vi "BNC555.ProcCases.vi"(0 "i ref in":refnum<vi>, 1 "selector":string, 2 "data":i8[](array[numeric]), 3 "call cluster":T1={"Object"="", "Selector"="", "CallType"=enum."synchronous", "Async Object"="", "Async Selector"="", "Data Descriptor"="", "Data"=[], "Error #"=0, "Expire"=0}, 5 "error in":errorcluster) -> (14 "i ref out":refnum<vi>, 17 "answer cluster":T1={"Object"="", "Selector"="", "CallType"=enum."synchronous", "Async Object"="", "Async Selector"="", "Data Descriptor"="", "Data"=[], "Error #"=0, "Expire"=0}, 19 "error out":errorcluster)   [LabVIEW 2014, in "BNC555.lvlib"]
doc: "This method is called by a process from within the default case in the event loop. The methods of a class that are linked to events will be called from THIS method. Add your code here."
uses:
  BNC555.lvlib
  CSCore/CSSystem/CoreDefs/CoreDefs.call_type.ctl
  CSCore/BaseProcess/BaseProcess.descriptor string definition.ctl
  CSCore/CSSystem/CoreDefs/CoreDefs.rawDataType.ctl
  CSCore/CSSystem/CoreLib/CoreLib.byte array 2 short.vi
  CSCore/CSSystem/CoreLib/CoreLib.string 2 byte array.vi
  CSCore/CSSystem/CoreLib/CoreLib.byte array 2 int.vi
  CSCore/CSSystem/CoreLib/CoreLib.byte array 2 double.vi
  CSCore/CSSystem/CoreLib/CoreLib.lvlib
  CSCore/BaseProcess/BaseProcess.lvlib
  non_GPL/instr.lib/BNC555/BNC555 - Driver np.lvlib
  CSCore/CAEObj/CAEObj.lvlib
  CSPhelix/PH_PSDBWriter/PH_PSDBWriter.lvlib
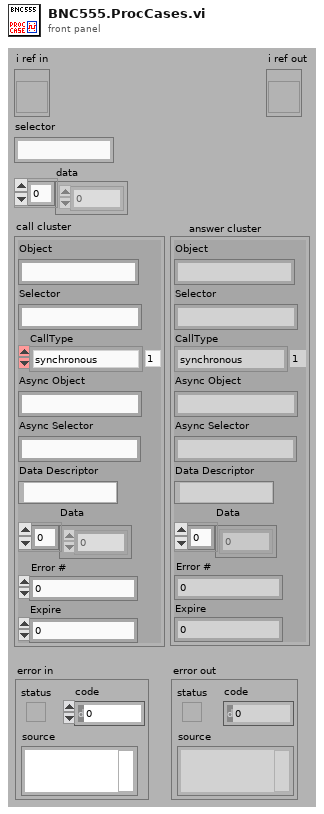
[diagram p1: front panel]
types:
  T1 = typedef "CoreDefs.call_type.ctl" = cluster{"Object":string, "Selector":string, "CallType":enum16{"simple", "synchronous", "asynchronous"}, "Async Object":string, "Async Selector":string, "Data Descriptor":T2, "Data":T3, "Error #":i32, "Expire":u32}
  T2 = typedef "BaseProcess.lvlib/BaseProcess.descriptor string definition.ctl" = string
  T3 = typedef "CoreDefs.rawDataType.ctl" = i8[]
  T4 = enum16{"All Info", "State", "Period", "Oscillator", "Mode", "Trigger"}
  T5 = enum16{"All Info", "State (On/Off)", "Output Config", "Mode Config", "Pulse Config", "Gate Config"}
  T6 = typedef "BNC555.lvlib/BNC555.i attribute.ctl" = cluster{"Information":cluster{"VISA resource name":refnum<visa-resource-name>, "Baud Rate (1:9600)":u16}, "Channel Array":T7[], "System":T8, "GUI Refs":cluster{"Delete":refnum<vi>, "Information":refnum<vi>, "System":refnum<vi>, "Channel Array":refnum<vi>, "Device Error":refnum<vi>, "Instr Driver Revision":refnum<vi>, "Instr Firmware Revision":refnum<vi>, "Instr Option":refnum<vi>, "Self-Test Response":refnum<vi>}, "Service IDs Channelinfo":i32[], "Service ID T0 Mode":i32}
  T7 = typedef "BNC555 - Driver np.lvlib/BNC555 All Chan Parameters.ctl" = cluster{"Chan #":i32, "Chan State":bool, "Chan Delay":dbl, "Chan Width":dbl, "Chan Mode":enum16{"Normal", "Single", "Burst", "Divide by N"}, "Chan Burst #":u32, "Chan Divide #":u32, "Chan Pol Out":enum16{"Normal", "Complement", "Inverted"}, "Chan Level Out":enum16{"TTL", "Adjustable", "35 Volt"}, "Chan Lev Adjust":dbl, "Chan Gate Pol":enum16{"Normal", "Complement", "Inverted"}, "Chan Gate State":bool}
  T8 = typedef "BNC555 - Driver np.lvlib/BNC555 All Sys Parameters.ctl" = cluster{"Sys Period":dbl, "Sys Oscillator":bool, "Sys Mode":enum16{"Normal", "Single", "Burst", "Duty Cycle"}, "Sys Burst #":u32, "Sys DC On":u32, "Sys DC Off":u32, "Sys Trig Mode":enum16{"Disabled", "Triggered", "Gated"}, "Sys Trig Lev":dbl, "Sys Gate State":bool, "Sys Trig Edge":bool, "Sys State":bool}
  T9 = typedef "PH_PSDBWriter.lvlib/PH_PSDBWriter.PHELIX-Subsystems.ctl" = i32
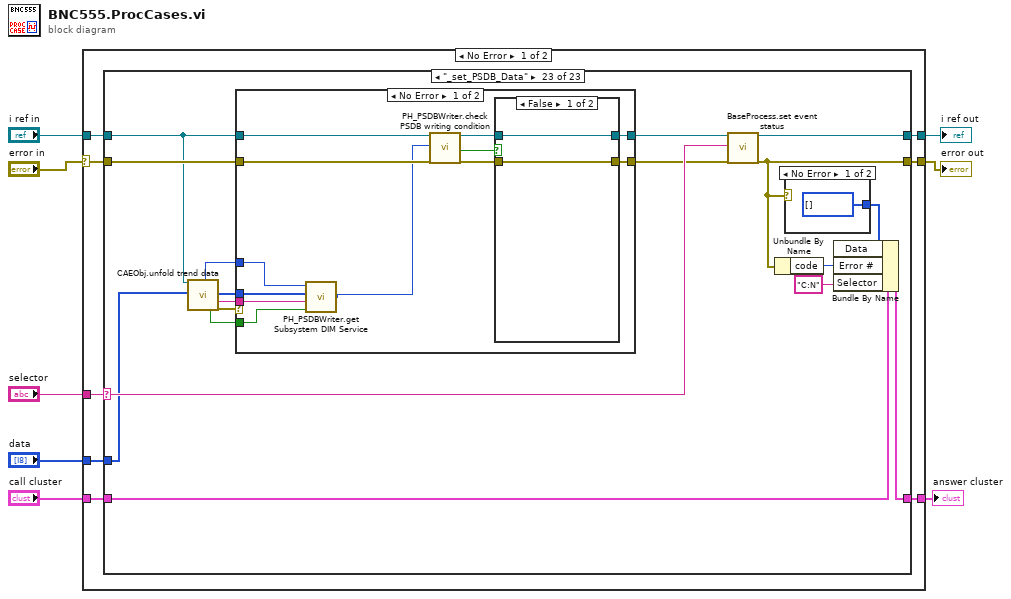
[diagram p0: block diagram]
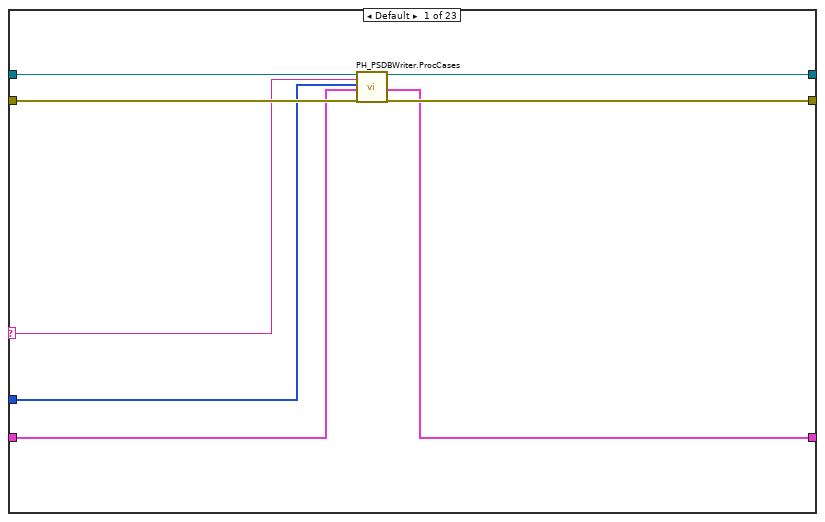
[diagram p2: hidden frame]
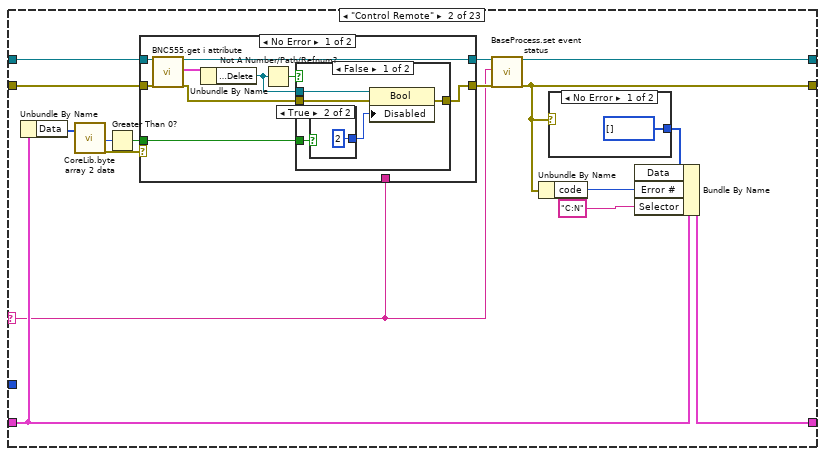
[diagram p3: hidden frame]
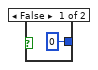
[diagram p4: hidden frame]
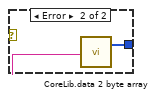
[diagram p7: hidden frame]
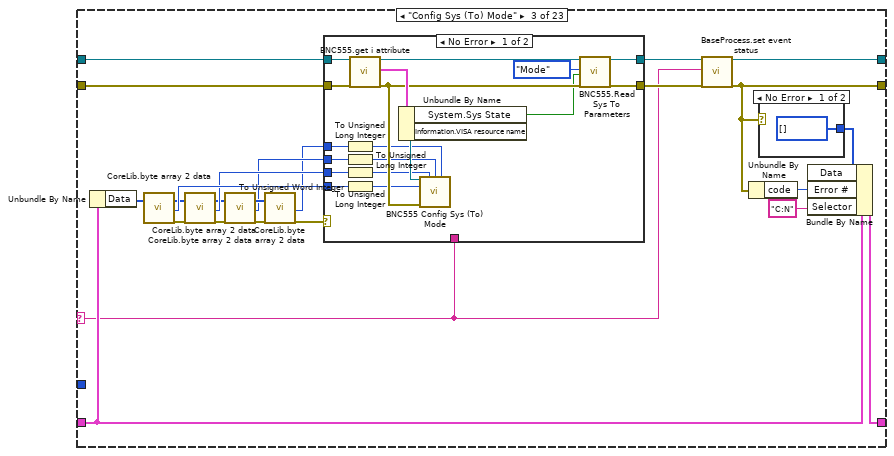
[diagram p8: hidden frame]
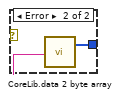
[diagram p10: hidden frame]
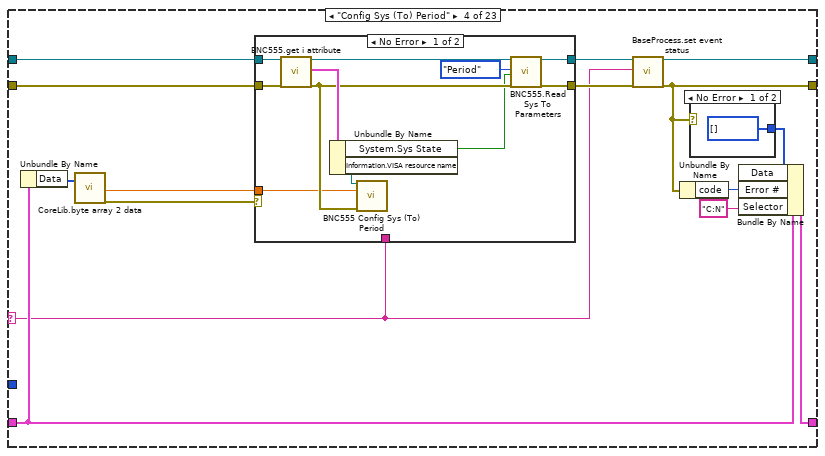
[diagram p11: hidden frame]
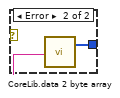
[diagram p13: hidden frame]
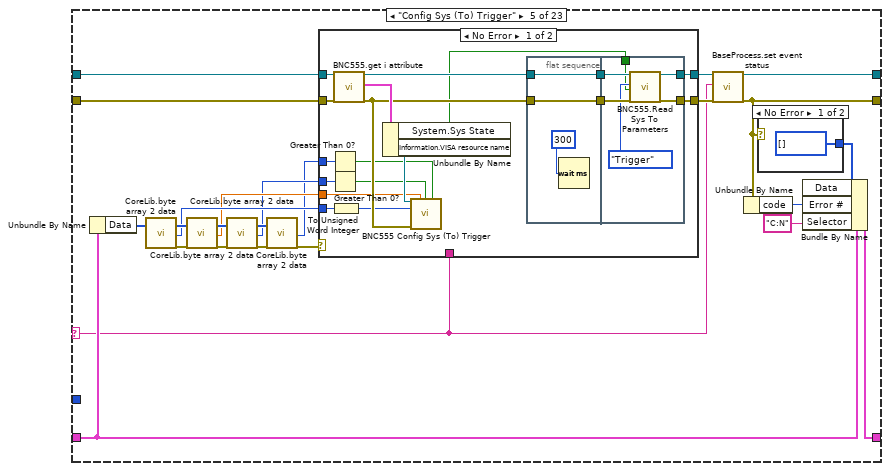
[diagram p14: hidden frame]
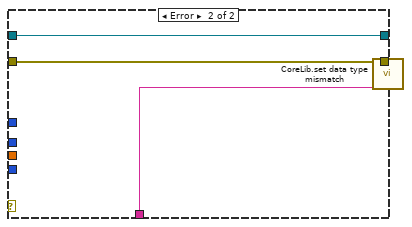
[diagram p15: hidden frame]
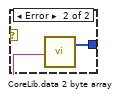
[diagram p16: hidden frame]
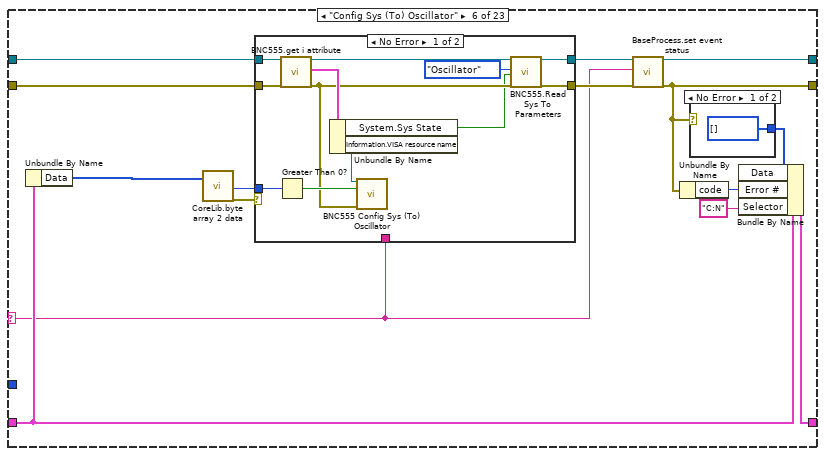
[diagram p17: hidden frame]
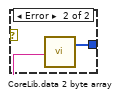
[diagram p19: hidden frame]
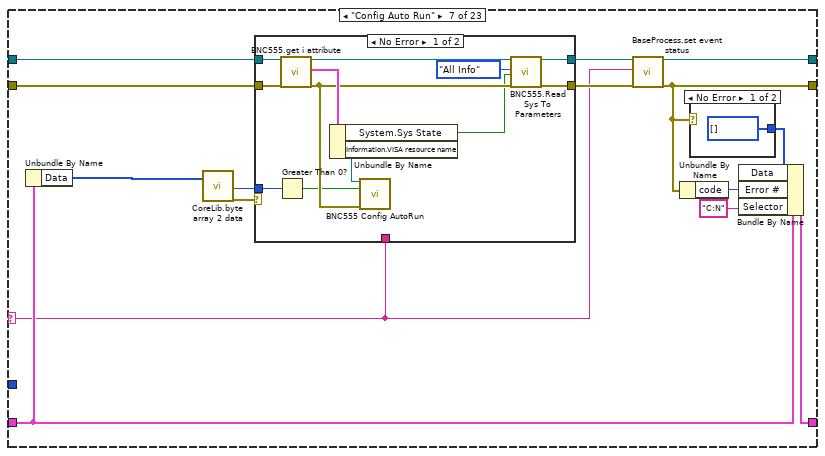
[diagram p20: hidden frame]
diagram:
  n1 = case shown="No Error" "error in" {
    selector: "error in" -> [w9 w806]
    tunnel: "selector" -> [w16 _]
    tunnel: [w15 w807] -> w7
    tunnel: "call cluster" -> [w14 w807]
    tunnel: "i ref in" -> [w13 w808]
    tunnel: [w12 w808] -> w4
    tunnel: [w11 w806] -> w3
    tunnel: "data" -> [w10 _]
    frame No Error {
      n2 = case shown="\"_set_PSDB_Data\"" w16 {
        selector: w16 -> [w19 w25 w77 w118 w162 w212 w247 w291 w333 w377 w421 w465 w503 w537 w560 w572 w610 w653 w681 w715 w731 w751 w773]
        tunnel: w13 -> [w18 w28 w80 w121 w165 w215 w250 w294 w336 w380 w424 w468 w506 w538 w556 w577 w615 w658 w685 w719 w735 w749 w765]
        tunnel: [w24 w38 w87 w128 w171 w221 w256 w300 w342 w386 w430 w474 w512 w544 w565 w587 w625 w662 w691 w723 w739 w755 w777] -> w12
        tunnel: w14 -> [w20 w30 w82 w123 w167 w217 w252 w296 w338 w382 w426 w470 w508 w540 w561 w575 w613 w656 w680 w714 w730 w750 w772]
        tunnel: [w21 w39 w88 w129 w172 w222 w257 w301 w343 w387 w431 w475 w513 w545 w566 w588 w626 w663 w692 w724 w740 w756 w778] -> w15
        tunnel: w9 -> [w23 w29 w81 w122 w166 w216 w251 w295 w337 w381 w425 w469 w507 w539 w554 w576 w614 w657 w684 w718 w734 w747 w766]
        tunnel: [w22 w36 w85 w126 w169 w219 w254 w298 w340 w384 w428 w472 w510 w542 w563 w585 w623 w660 w689 w721 w737 w753 w775] -> w11
        tunnel: w10 -> [w17 _ _ _ _ _ _ _ _ _ _ _ _ _ _ _ _ _ _ _ _ _ w762]
        frame Default {
          # "In the default case, always call the ProcCase method of the parent class"
          n3 = call "PH_PSDBWriter.ProcCases.vi"("i ref in"=w18, "selector"=w19, "Data"=w17, "call cluster"=w20, "error in"=w23) -> ("i ref out"=w24:refnum<vi>, "answer cluster"=w21:T1, "error out"=w22:errorcluster)  [unwired: 12 in]
        }
        frame "Control Remote" {
          n4 = Unbundle By Name(w30) -> ("Data"=w31:T3)
          n5 = call-poly "CoreLib.byte array 2 data.vi"("byteArray"=w31) -> ("i16"=w32:i16, "error out"=w34:errorcluster)  [unwired: 16 in, 1 out]
          n6 = Greater Than 0?(x=w32) -> (x > 0?=w33:bool)
          n7 = case shown="No Error" w34 {
            tunnel: [w43 w61] -> w26
            tunnel: w28 -> [w49 w61]
            tunnel: w29 -> [w48 w60]
            tunnel: [w44 w59] -> w27
            tunnel: w25 -> [_ w58]
            tunnel: w33 -> [w45 _]
            frame No Error {
              n8 = call "BNC555.get i attribute.vi"("i ref in"=w49, "error in (no error)"=w48) -> ("i ref out"=w43:refnum<vi>, "i attribute"=w47:T6, "error out"=w46:errorcluster)  [unwired: 15 in]
              n9 = Unbundle By Name(w47) -> ("GUI Refs.Delete"=w42:refnum<vi>)
              n10 = Not A Number/Path/Refnum?(number/path/refnum=w42) -> (NaN/Path/Refnum?=w41:bool)
              n11 = case shown="False" w41 {
                tunnel: w42 -> [w54 _]
                tunnel: w46 -> [w53 w57]
                tunnel: [w52 w57] -> w44
                tunnel: w45 -> [w51 _]
                frame False {
                  n12 = case shown="True" w51 {
                    tunnel: [0 2] -> w50
                    frame False {
                    }
                    frame True {
                    }
                  }
                  n13 = property class="Bool"(reference=w54, error in=w53, "Disabled"=w50) -> (error out=w52:errorcluster)  [unwired: 1 out]
                }
                frame True {
                }
              }
            }
            frame Error {
              n14 = call "CoreLib.set data type mismatch.vi"("error in (no error)"=w60, "error source"=w58) -> ("error out"=w59:errorcluster)  [unwired: 17 in]
            }
          }
          n15 = call "BaseProcess.set event status.vi"("i ref in"=w26, "EventStatus"=w25, "error in (no error)"=w27) -> ("i ref out"=w38:refnum<vi>, "error out"=w36:errorcluster)  [unwired: 14 in, 1 out]
          n16 = Unbundle By Name(w36) -> ("code"=w40:i32)
          n17 = case shown="No Error" w36 {
            selector: w36 -> [_ w65]
            tunnel: [T3 [] ("byteArray out") w63] -> w37
            frame No Error {
            }
            frame Error {
              n18 = Unbundle By Name(w65) -> ("source"=w64:string)
              n19 = call-poly "CoreLib.data 2 byte array.vi"("string"=w64) -> ("byteArray out"=w63:T3)  [unwired: 18 in]
            }
          }
          n20 = Bundle By Name(cluster=w30, "Data"=w37, "Error #"=w40, "Selector"="C:N") -> (w39:T1)
        }
        frame "Config Sys (To) Mode" {
          n21 = Unbundle By Name(w82) -> ("Data"=w83:T3)
          n22 = call-poly "CoreLib.byte array 2 data.vi"("byteArray"=w83) -> ("byteArray out"=w70:T3, "i16"=w76:i16, "error out"=w75:errorcluster)  [unwired: 16 in]
          n23 = call-poly "CoreLib.byte array 2 data.vi"("byteArray"=w70, "error in (no error)"=w75) -> ("byteArray out"=w69:T3, "i32"=w71:i32, "error out"=w74:errorcluster)  [unwired: 15 in]
          n24 = call-poly "CoreLib.byte array 2 data.vi"("byteArray"=w69, "error in (no error)"=w74) -> ("byteArray out"=w68:T3, "i32"=w67:i32, "error out"=w73:errorcluster)  [unwired: 15 in]
          n25 = call-poly "CoreLib.byte array 2 data.vi"("byteArray"=w68, "error in (no error)"=w73) -> ("i32"=w66:i32, "error out"=w72:errorcluster)  [unwired: 15 in, 1 out]
          n26 = case shown="No Error" w72 {
            tunnel: [w102 w111] -> w78
            tunnel: w80 -> [w107 w111]
            tunnel: w81 -> [w106 w110]
            tunnel: [w100 w109] -> w79
            tunnel: w77 -> [_ w108]
            tunnel: w76 -> [w99 _]
            tunnel: w71 -> [w97 _]
            tunnel: w67 -> [w96 _]
            tunnel: w66 -> [w93 _]
            frame No Error {
              n27 = To Unsigned Long Integer(number=w93) -> (unsigned 32bit integer=w92:u32)
              n28 = To Unsigned Long Integer(number=w96) -> (unsigned 32bit integer=w94:u32)
              n29 = To Unsigned Long Integer(number=w97) -> (unsigned 32bit integer=w95:u32)
              n30 = To Unsigned Word Integer(number=w99) -> (unsigned 16bit integer=w98:u16)
              n31 = call "BNC555.get i attribute.vi"("i ref in"=w107, "error in (no error)"=w106) -> ("i ref out"=w103:refnum<vi>, "i attribute"=w105:T6, "error out"=w101:errorcluster)  [unwired: 15 in]
              n32 = Unbundle By Name(w105) -> ("System.Sys State"=w90:bool, "Information.VISA resource name"=w104:refnum<visa-resource-name>)
              n33 = call "BNC555 Config Sys (To) Mode.vi"("VISA resource"=w104, "Burst # (10)"=w95, "DC On (10)"=w94, "DC Off (10)"=w92, "Mode (0:Normal)"=w98, "error in (no error)"=w101) -> ()  [unwired: 8 in, 2 out]
              n34 = call "BNC555.Read Sys To Parameters.vi"("i ref in"=w103, "Parameter"=T4."Mode", "Sys State"=w90, "error in (no error)"=w101) -> ("i ref out"=w102:refnum<vi>, "error out"=w100:errorcluster)  [unwired: 14 in]
            }
            frame Error {
              n35 = call "CoreLib.set data type mismatch.vi"("error in (no error)"=w110, "error source"=w108) -> ("error out"=w109:errorcluster)  [unwired: 17 in]
            }
          }
          n36 = call "BaseProcess.set event status.vi"("i ref in"=w78, "EventStatus"=w77, "error in (no error)"=w79) -> ("i ref out"=w87:refnum<vi>, "error out"=w85:errorcluster)  [unwired: 14 in, 1 out]
          n37 = Unbundle By Name(w85) -> ("code"=w89:i32)
          n38 = case shown="No Error" w85 {
            selector: w85 -> [_ w115]
            tunnel: [T3 [] ("byteArray out") w113] -> w86
            frame No Error {
            }
            frame Error {
              n39 = Unbundle By Name(w115) -> ("source"=w114:string)
              n40 = call-poly "CoreLib.data 2 byte array.vi"("string"=w114) -> ("byteArray out"=w113:T3)  [unwired: 18 in]
            }
          }
          n41 = Bundle By Name(cluster=w82, "Data"=w86, "Error #"=w89, "Selector"="C:N") -> (w88:T1)
        }
        frame "Config Sys (To) Period" {
          n42 = Unbundle By Name(w123) -> ("Data"=w124:T3)
          n43 = call-poly "CoreLib.byte array 2 data.vi"("byteArray"=w124) -> ("d64"=w117:dbl, "error out"=w116:errorcluster)  [unwired: 16 in, 1 out]
          n44 = case shown="No Error" w116 {
            tunnel: [w137 w145] -> w119
            tunnel: w121 -> [w141 w145]
            tunnel: w122 -> [w140 w144]
            tunnel: [w136 w143] -> w120
            tunnel: w118 -> [_ w142]
            tunnel: w117 -> [w134 _]
            frame No Error {
              n45 = call "BNC555.get i attribute.vi"("i ref in"=w141, "error in (no error)"=w140) -> ("i ref out"=w138:refnum<vi>, "i attribute"=w139:T6, "error out"=w135:errorcluster)  [unwired: 15 in]
              n46 = Unbundle By Name(w139) -> ("System.Sys State"=w131:bool, "Information.VISA resource name"=w133:refnum<visa-resource-name>)
              n47 = call "BNC555 Config Sys (To) Period.vi"("VISA resource"=w133, "Period (100 msec)"=w134, "error in (no error)"=w135) -> ()  [unwired: 11 in, 2 out]
              n48 = call "BNC555.Read Sys To Parameters.vi"("i ref in"=w138, "Parameter"=T4."Period", "Sys State"=w131, "error in (no error)"=w135) -> ("i ref out"=w137:refnum<vi>, "error out"=w136:errorcluster)  [unwired: 14 in]
            }
            frame Error {
              n49 = call "CoreLib.set data type mismatch.vi"("error in (no error)"=w144, "error source"=w142) -> ("error out"=w143:errorcluster)  [unwired: 17 in]
            }
          }
          n50 = call "BaseProcess.set event status.vi"("i ref in"=w119, "EventStatus"=w118, "error in (no error)"=w120) -> ("i ref out"=w128:refnum<vi>, "error out"=w126:errorcluster)  [unwired: 14 in, 1 out]
          n51 = Unbundle By Name(w126) -> ("code"=w130:i32)
          n52 = case shown="No Error" w126 {
            selector: w126 -> [_ w149]
            tunnel: [T3 [] ("byteArray out") w147] -> w127
            frame No Error {
            }
            frame Error {
              n53 = Unbundle By Name(w149) -> ("source"=w148:string)
              n54 = call-poly "CoreLib.data 2 byte array.vi"("string"=w148) -> ("byteArray out"=w147:T3)  [unwired: 18 in]
            }
          }
          n55 = Bundle By Name(cluster=w123, "Data"=w127, "Error #"=w130, "Selector"="C:N") -> (w129:T1)
        }
        frame "Config Sys (To) Trigger" {
          n56 = Unbundle By Name(w167) -> ("Data"=w155:T3)
          n57 = call-poly "CoreLib.byte array 2 data.vi"("byteArray"=w155) -> ("byteArray out"=w158:T3, "i16"=w153:i16, "error out"=w161:errorcluster)  [unwired: 16 in]
          n58 = call-poly "CoreLib.byte array 2 data.vi"("byteArray"=w158, "error in (no error)"=w161) -> ("byteArray out"=w157:T3, "d64"=w152:dbl, "error out"=w160:errorcluster)  [unwired: 15 in]
          n59 = call-poly "CoreLib.byte array 2 data.vi"("byteArray"=w157, "error in (no error)"=w160) -> ("byteArray out"=w156:T3, "i16"=w151:i16, "error out"=w159:errorcluster)  [unwired: 15 in]
          n60 = call-poly "CoreLib.byte array 2 data.vi"("byteArray"=w156, "error in (no error)"=w159) -> ("i16"=w150:i16, "error out"=w154:errorcluster)  [unwired: 15 in, 1 out]
          n61 = case shown="No Error" w154 {
            tunnel: [w187 w204] -> w163
            tunnel: w165 -> [w191 w204]
            tunnel: w166 -> [w190 w203]
            tunnel: [w186 w202] -> w164
            tunnel: w162 -> [_ w201]
            tunnel: w153 -> [w182 _]
            tunnel: w152 -> [w179 _]
            tunnel: w151 -> [w181 _]
            tunnel: w150 -> [w178 _]
            frame No Error {
              n62 = Greater Than 0?(x=w178) -> (x > 0?=w177:bool)
              n63 = Greater Than 0?(x=w181) -> (x > 0?=w180:bool)
              n64 = To Unsigned Word Integer(number=w182) -> (unsigned 16bit integer=w183:u16)
              n65 = call "BNC555.get i attribute.vi"("i ref in"=w191, "error in (no error)"=w190) -> ("i ref out"=w188:refnum<vi>, "i attribute"=w189:T6, "error out"=w185:errorcluster)  [unwired: 15 in]
              n66 = Unbundle By Name(w189) -> ("System.Sys State"=w174:bool, "Information.VISA resource name"=w184:refnum<visa-resource-name>)
              n67 = call "BNC555 Config Sys (To) Trigger.vi"("VISA resource"=w184, "Trigger Level (2.5V)"=w179, "Trigger Edge (T:Rising)"=w180, "Gate Polarity (T:High)"=w177, "Mode (0:Disabled)"=w183, "error in (no error)"=w185) -> ()  [unwired: 8 in, 2 out]
              n68 = flat-sequence {
                tunnel: w185 -> [w193]
                tunnel: w188 -> [w194]
                tunnel: [w194] -> w176
                tunnel: [w193] -> w175
                tunnel: [w199] -> w187
                tunnel: [w198] -> w186
                tunnel: w176 -> [w200]
                tunnel: w175 -> [w197]
                tunnel: w174 -> [w195]
                frame #0 {
                  n69 = Wait (ms)(milliseconds to wait=u32 300) -> ()  [unwired: 1 out]
                }
                frame #1 {
                  n70 = call "BNC555.Read Sys To Parameters.vi"("i ref in"=w200, "Parameter"=T4."Trigger", "Sys State"=w195, "error in (no error)"=w197) -> ("i ref out"=w199:refnum<vi>, "error out"=w198:errorcluster)  [unwired: 14 in]
                }
              }
            }
            frame Error {
              n71 = call "CoreLib.set data type mismatch.vi"("error in (no error)"=w203, "error source"=w201) -> ("error out"=w202:errorcluster)  [unwired: 17 in]
            }
          }
          n72 = call "BaseProcess.set event status.vi"("i ref in"=w163, "EventStatus"=w162, "error in (no error)"=w164) -> ("i ref out"=w171:refnum<vi>, "error out"=w169:errorcluster)  [unwired: 14 in, 1 out]
          n73 = Unbundle By Name(w169) -> ("code"=w173:i32)
          n74 = case shown="No Error" w169 {
            selector: w169 -> [_ w208]
            tunnel: [T3 [] ("byteArray out") w206] -> w170
            frame No Error {
            }
            frame Error {
              n75 = Unbundle By Name(w208) -> ("source"=w207:string)
              n76 = call-poly "CoreLib.data 2 byte array.vi"("string"=w207) -> ("byteArray out"=w206:T3)  [unwired: 18 in]
            }
          }
          n77 = Bundle By Name(cluster=w167, "Data"=w170, "Error #"=w173, "Selector"="C:N") -> (w172:T1)
        }
        frame "Config Sys (To) Oscillator" {
          n78 = Unbundle By Name(w217) -> ("Data"=w209:T3)
          n79 = call-poly "CoreLib.byte array 2 data.vi"("byteArray"=w209) -> ("i16"=w210:i16, "error out"=w211:errorcluster)  [unwired: 16 in, 1 out]
          n80 = case shown="No Error" w211 {
            tunnel: [w231 w239] -> w213
            tunnel: w215 -> [w235 w239]
            tunnel: w216 -> [w234 w238]
            tunnel: [w230 w237] -> w214
            tunnel: w212 -> [_ w236]
            tunnel: w210 -> [w229 _]
            frame No Error {
              n81 = Greater Than 0?(x=w229) -> (x > 0?=w228:bool)
              n82 = call "BNC555.get i attribute.vi"("i ref in"=w235, "error in (no error)"=w234) -> ("i ref out"=w232:refnum<vi>, "i attribute"=w233:T6, "error out"=w226:errorcluster)  [unwired: 15 in]
              n83 = Unbundle By Name(w233) -> ("System.Sys State"=w224:bool, "Information.VISA resource name"=w227:refnum<visa-resource-name>)
              n84 = call "BNC555 Config Sys (To) Oscillator.vi"("VISA resource"=w227, "Oscillator (F:Internal)"=w228, "error in (no error)"=w226) -> ()  [unwired: 11 in, 2 out]
              n85 = call "BNC555.Read Sys To Parameters.vi"("i ref in"=w232, "Parameter"=T4."Oscillator", "Sys State"=w224, "error in (no error)"=w226) -> ("i ref out"=w231:refnum<vi>, "error out"=w230:errorcluster)  [unwired: 14 in]
            }
            frame Error {
              n86 = call "CoreLib.set data type mismatch.vi"("error in (no error)"=w238, "error source"=w236) -> ("error out"=w237:errorcluster)  [unwired: 17 in]
            }
          }
          n87 = call "BaseProcess.set event status.vi"("i ref in"=w213, "EventStatus"=w212, "error in (no error)"=w214) -> ("i ref out"=w221:refnum<vi>, "error out"=w219:errorcluster)  [unwired: 14 in, 1 out]
          n88 = Unbundle By Name(w219) -> ("code"=w223:i32)
          n89 = case shown="No Error" w219 {
            selector: w219 -> [_ w243]
            tunnel: [T3 [] ("byteArray out") w241] -> w220
            frame No Error {
            }
            frame Error {
              n90 = Unbundle By Name(w243) -> ("source"=w242:string)
              n91 = call-poly "CoreLib.data 2 byte array.vi"("string"=w242) -> ("byteArray out"=w241:T3)  [unwired: 18 in]
            }
          }
          n92 = Bundle By Name(cluster=w217, "Data"=w220, "Error #"=w223, "Selector"="C:N") -> (w222:T1)
        }
        frame "Config Auto Run" {
          n93 = Unbundle By Name(w252) -> ("Data"=w244:T3)
          n94 = call-poly "CoreLib.byte array 2 data.vi"("byteArray"=w244) -> ("i16"=w245:i16, "error out"=w246:errorcluster)  [unwired: 16 in, 1 out]
          n95 = case shown="No Error" w246 {
            tunnel: [w266 w274] -> w248
            tunnel: w250 -> [w270 w274]
            tunnel: w251 -> [w269 w273]
            tunnel: [w265 w272] -> w249
            tunnel: w247 -> [_ w271]
            tunnel: w245 -> [w264 _]
            frame No Error {
              n96 = Greater Than 0?(x=w264) -> (x > 0?=w261:bool)
              n97 = call "BNC555.get i attribute.vi"("i ref in"=w270, "error in (no error)"=w269) -> ("i ref out"=w267:refnum<vi>, "i attribute"=w268:T6, "error out"=w262:errorcluster)  [unwired: 15 in]
              n98 = Unbundle By Name(w268) -> ("System.Sys State"=w259:bool, "Information.VISA resource name"=w263:refnum<visa-resource-name>)
              n99 = call "BNC555 Config AutoRun.vi"("VISA resource"=w263, "AutoRun (F:Disabled)"=w261, "error in (no error)"=w262) -> ()  [unwired: 11 in, 2 out]
              n100 = call "BNC555.Read Sys To Parameters.vi"("i ref in"=w267, "Parameter"=T4."All Info", "Sys State"=w259, "error in (no error)"=w262) -> ("i ref out"=w266:refnum<vi>, "error out"=w265:errorcluster)  [unwired: 14 in]
            }
            frame Error {
              n101 = call "CoreLib.set data type mismatch.vi"("error in (no error)"=w273, "error source"=w271) -> ("error out"=w272:errorcluster)  [unwired: 17 in]
            }
          }
          n102 = call "BaseProcess.set event status.vi"("i ref in"=w248, "EventStatus"=w247, "error in (no error)"=w249) -> ("i ref out"=w256:refnum<vi>, "error out"=w254:errorcluster)  [unwired: 14 in, 1 out]
          n103 = Unbundle By Name(w254) -> ("code"=w258:i32)
          n104 = case shown="No Error" w254 {
            selector: w254 -> [_ w278]
            tunnel: [T3 [] ("byteArray out") w276] -> w255
            frame No Error {
            }
            frame Error {
              n105 = Unbundle By Name(w278) -> ("source"=w277:string)
              n106 = call-poly "CoreLib.data 2 byte array.vi"("string"=w277) -> ("byteArray out"=w276:T3)  [unwired: 18 in]
            }
          }
          n107 = Bundle By Name(cluster=w252, "Data"=w255, "Error #"=w258, "Selector"="C:N") -> (w257:T1)
        }
        frame "Config Chan Mode" {
          n108 = Unbundle By Name(w296) -> ("Data"=w290:T3)
          n109 = call-poly "CoreLib.byte array 2 data.vi"("byteArray"=w290) -> ("byteArray out"=w286:T3, "i32"=w289:i32, "error out"=w288:errorcluster)  [unwired: 16 in]
          n110 = call-poly "CoreLib.byte array 2 data.vi"("byteArray"=w286, "error in (no error)"=w288) -> ("byteArray out"=w282:T3, "i16"=w287:i16, "error out"=w284:errorcluster)  [unwired: 15 in]
          n111 = call-poly "CoreLib.byte array 2 data.vi"("byteArray"=w282, "error in (no error)"=w284) -> ("byteArray out"=w281:T3, "i32"=w280:i32, "error out"=w285:errorcluster)  [unwired: 15 in]
          n112 = call-poly "CoreLib.byte array 2 data.vi"("byteArray"=w281, "error in (no error)"=w285) -> ("i32"=w279:i32, "error out"=w283:errorcluster)  [unwired: 15 in, 1 out]
          n113 = case shown="No Error" w283 {
            tunnel: [w314 w322] -> w292
            tunnel: w294 -> [w318 w322]
            tunnel: w295 -> [w317 w321]
            tunnel: [w313 w320] -> w293
            tunnel: w291 -> [_ w319]
            tunnel: w289 -> [w310 _]
            tunnel: w287 -> [w308 _]
            tunnel: w280 -> [w305 _]
            tunnel: w279 -> [w304 _]
            frame No Error {
              n114 = call "BNC555.get i attribute.vi"("i ref in"=w318, "error in (no error)"=w317) -> ("i ref out"=w315:refnum<vi>, "i attribute"=w316:T6, "error out"=w311:errorcluster)  [unwired: 15 in]
              n115 = Unbundle By Name(w316) -> ("Information.VISA resource name"=w312:refnum<visa-resource-name>)
              n116 = To Unsigned Long Integer(number=w305) -> (unsigned 32bit integer=w306:u32)
              n117 = To Unsigned Long Integer(number=w304) -> (unsigned 32bit integer=w307:u32)
              n118 = To Unsigned Word Integer(number=w308) -> (unsigned 16bit integer=w309:u16)
              n119 = call "BNC555 Config Chan Mode.vi"("VISA resource"=w312, "Burst # (10)"=w307, "Divide # (10)"=w306, "Channel (1:Chan A)"=w310, "Mode (0:Normal)"=w309, "error in (no error)"=w311) -> ()  [unwired: 8 in, 2 out]
              n120 = call "BNC555.Read Channel Parameters.vi"("i ref in"=w315, "Channel (1: Chan A)"=w310, "Parameter"=T5."Mode Config", "error in (no error)"=w311) -> ("i ref out"=w314:refnum<vi>, "error out"=w313:errorcluster)  [unwired: 14 in]
            }
            frame Error {
              n121 = call "CoreLib.set data type mismatch.vi"("error in (no error)"=w321, "error source"=w319) -> ("error out"=w320:errorcluster)  [unwired: 17 in]
            }
          }
          n122 = call "BaseProcess.set event status.vi"("i ref in"=w292, "EventStatus"=w291, "error in (no error)"=w293) -> ("i ref out"=w300:refnum<vi>, "error out"=w298:errorcluster)  [unwired: 14 in, 1 out]
          n123 = Unbundle By Name(w298) -> ("code"=w302:i32)
          n124 = case shown="No Error" w298 {
            selector: w298 -> [_ w326]
            tunnel: [T3 [] ("byteArray out") w324] -> w299
            frame No Error {
            }
            frame Error {
              n125 = Unbundle By Name(w326) -> ("source"=w325:string)
              n126 = call-poly "CoreLib.data 2 byte array.vi"("string"=w325) -> ("byteArray out"=w324:T3)  [unwired: 18 in]
            }
          }
          n127 = Bundle By Name(cluster=w296, "Data"=w299, "Error #"=w302, "Selector"="C:N") -> (w301:T1)
        }
        frame "Config Chan Gating" {
          n128 = Unbundle By Name(w338) -> ("Data"=w332:T3)
          n129 = call-poly "CoreLib.byte array 2 data.vi"("byteArray"=w332) -> ("byteArray out"=w328:T3, "i32"=w331:i32, "error out"=w330:errorcluster)  [unwired: 16 in]
          n130 = call-poly "CoreLib.byte array 2 data.vi"("byteArray"=w328, "error in (no error)"=w330) -> ("i16"=w329:i16, "error out"=w327:errorcluster)  [unwired: 15 in, 1 out]
          n131 = case shown="No Error" w327 {
            tunnel: [w352 w360] -> w334
            tunnel: w336 -> [w356 w360]
            tunnel: w337 -> [w355 w359]
            tunnel: [w351 w358] -> w335
            tunnel: w333 -> [_ w357]
            tunnel: w331 -> [w347 _]
            tunnel: w329 -> [w350 _]
            frame No Error {
              n132 = call "BNC555.get i attribute.vi"("i ref in"=w356, "error in (no error)"=w355) -> ("i ref out"=w353:refnum<vi>, "i attribute"=w354:T6, "error out"=w349:errorcluster)  [unwired: 15 in]
              n133 = Unbundle By Name(w354) -> ("Information.VISA resource name"=w348:refnum<visa-resource-name>)
              n134 = To Unsigned Word Integer(number=w350) -> (unsigned 16bit integer=w346:u16)
              n135 = call "BNC555 Config Chan Gating.vi"("VISA resource"=w348, "Channel (1:Chan A)"=w347, "Polarity (Normal)"=w346, "error in (no error)"=w349) -> ()  [unwired: 10 in, 2 out]
              n136 = call "BNC555.Read Channel Parameters.vi"("i ref in"=w353, "Channel (1: Chan A)"=w347, "Parameter"=T5."Gate Config", "error in (no error)"=w349) -> ("i ref out"=w352:refnum<vi>, "error out"=w351:errorcluster)  [unwired: 14 in]
            }
            frame Error {
              n137 = call "CoreLib.set data type mismatch.vi"("error in (no error)"=w359, "error source"=w357) -> ("error out"=w358:errorcluster)  [unwired: 17 in]
            }
          }
          n138 = call "BaseProcess.set event status.vi"("i ref in"=w334, "EventStatus"=w333, "error in (no error)"=w335) -> ("i ref out"=w342:refnum<vi>, "error out"=w340:errorcluster)  [unwired: 14 in, 1 out]
          n139 = Unbundle By Name(w340) -> ("code"=w344:i32)
          n140 = case shown="No Error" w340 {
            selector: w340 -> [_ w364]
            tunnel: [T3 [] ("byteArray out") w362] -> w341
            frame No Error {
            }
            frame Error {
              n141 = Unbundle By Name(w364) -> ("source"=w363:string)
              n142 = call-poly "CoreLib.data 2 byte array.vi"("string"=w363) -> ("byteArray out"=w362:T3)  [unwired: 18 in]
            }
          }
          n143 = Bundle By Name(cluster=w338, "Data"=w341, "Error #"=w344, "Selector"="C:N") -> (w343:T1)
        }
        frame "Config Chan Output" {
          n144 = Unbundle By Name(w382) -> ("Data"=w376:T3)
          n145 = call-poly "CoreLib.byte array 2 data.vi"("byteArray"=w376) -> ("byteArray out"=w372:T3, "i32"=w375:i32, "error out"=w374:errorcluster)  [unwired: 16 in]
          n146 = call-poly "CoreLib.byte array 2 data.vi"("byteArray"=w372, "error in (no error)"=w374) -> ("byteArray out"=w370:T3, "i16"=w373:i16, "error out"=w371:errorcluster)  [unwired: 15 in]
          n147 = call-poly "CoreLib.byte array 2 data.vi"("byteArray"=w370, "error in (no error)"=w371) -> ("byteArray out"=w366:T3, "i16"=w369:i16, "error out"=w368:errorcluster)  [unwired: 15 in]
          n148 = call-poly "CoreLib.byte array 2 data.vi"("byteArray"=w366, "error in (no error)"=w368) -> ("d64"=w365:dbl, "error out"=w367:errorcluster)  [unwired: 15 in, 1 out]
          n149 = case shown="No Error" w367 {
            tunnel: [w390 w407] -> w378
            tunnel: w380 -> [w403 w407]
            tunnel: w381 -> [w402 w406]
            tunnel: [w389 w405] -> w379
            tunnel: w377 -> [_ w404]
            tunnel: w375 -> [w392 _]
            tunnel: w373 -> [w399 _]
            tunnel: w369 -> [w395 _]
            tunnel: w365 -> [w393 _]
            frame No Error {
              n150 = To Unsigned Word Integer(number=w395) -> (unsigned 16bit integer=w394:u16)
              n151 = To Unsigned Word Integer(number=w399) -> (unsigned 16bit integer=w396:u16)
              n152 = call "BNC555.get i attribute.vi"("i ref in"=w403, "error in (no error)"=w402) -> ("i ref out"=w400:refnum<vi>, "i attribute"=w401:T6, "error out"=w398:errorcluster)  [unwired: 15 in]
              n153 = Unbundle By Name(w401) -> ("Information.VISA resource name"=w397:refnum<visa-resource-name>)
              n154 = call "BNC555 Config Chan Output.vi"("VISA resource"=w397, "Polarity (Normal)"=w396, "Level (TTL)"=w394, "Adjustable (5 Volts)"=w393, "Channel (1:Chan A)"=w392, "error in (no error)"=w398) -> ()  [unwired: 8 in, 2 out]
              n155 = call "BNC555.Read Channel Parameters.vi"("i ref in"=w400, "Channel (1: Chan A)"=w392, "Parameter"=T5."Output Config", "error in (no error)"=w398) -> ("i ref out"=w390:refnum<vi>, "error out"=w389:errorcluster)  [unwired: 14 in]
            }
            frame Error {
              n156 = call "CoreLib.set data type mismatch.vi"("error in (no error)"=w406, "error source"=w404) -> ("error out"=w405:errorcluster)  [unwired: 17 in]
            }
          }
          n157 = call "BaseProcess.set event status.vi"("i ref in"=w378, "EventStatus"=w377, "error in (no error)"=w379) -> ("i ref out"=w386:refnum<vi>, "error out"=w384:errorcluster)  [unwired: 14 in, 1 out]
          n158 = Unbundle By Name(w384) -> ("code"=w388:i32)
          n159 = case shown="No Error" w384 {
            selector: w384 -> [_ w411]
            tunnel: [T3 [] ("byteArray out") w409] -> w385
            frame No Error {
            }
            frame Error {
              n160 = Unbundle By Name(w411) -> ("source"=w410:string)
              n161 = call-poly "CoreLib.data 2 byte array.vi"("string"=w410) -> ("byteArray out"=w409:T3)  [unwired: 18 in]
            }
          }
          n162 = Bundle By Name(cluster=w382, "Data"=w385, "Error #"=w388, "Selector"="C:N") -> (w387:T1)
        }
        frame "Config Chan Pulse" {
          n163 = Unbundle By Name(w426) -> ("Data"=w420:T3)
          n164 = call-poly "CoreLib.byte array 2 data.vi"("byteArray"=w420) -> ("byteArray out"=w416:T3, "i32"=w419:i32, "error out"=w418:errorcluster)  [unwired: 16 in]
          n165 = call-poly "CoreLib.byte array 2 data.vi"("byteArray"=w416, "error in (no error)"=w418) -> ("byteArray out"=w412:T3, "d64"=w417:dbl, "error out"=w413:errorcluster)  [unwired: 15 in]
          n166 = call-poly "CoreLib.byte array 2 data.vi"("byteArray"=w412, "error in (no error)"=w413) -> ("d64"=w414:dbl, "error out"=w415:errorcluster)  [unwired: 15 in, 1 out]
          n167 = case shown="No Error" w415 {
            tunnel: [w440 w448] -> w422
            tunnel: w424 -> [w444 w448]
            tunnel: w425 -> [w443 w447]
            tunnel: [w439 w446] -> w423
            tunnel: w421 -> [_ w445]
            tunnel: w419 -> [w437 _]
            tunnel: w417 -> [w434 _]
            tunnel: w414 -> [w435 _]
            frame No Error {
              n168 = call "BNC555.get i attribute.vi"("i ref in"=w444, "error in (no error)"=w443) -> ("i ref out"=w441:refnum<vi>, "i attribute"=w442:T6, "error out"=w438:errorcluster)  [unwired: 15 in]
              n169 = Unbundle By Name(w442) -> ("Information.VISA resource name"=w436:refnum<visa-resource-name>)
              n170 = call "BNC555 Config Chan Pulse.vi"("VISA resource"=w436, "Delay (10 msec)"=w434, "Width (10 msec)"=w435, "Channel (1:Chan A)"=w437, "error in (no error)"=w438) -> ()  [unwired: 9 in, 2 out]
              n171 = call "BNC555.Read Channel Parameters.vi"("i ref in"=w441, "Channel (1: Chan A)"=w437, "Parameter"=T5."Pulse Config", "error in (no error)"=w438) -> ("i ref out"=w440:refnum<vi>, "error out"=w439:errorcluster)  [unwired: 14 in]
            }
            frame Error {
              n172 = call "CoreLib.set data type mismatch.vi"("error in (no error)"=w447, "error source"=w445) -> ("error out"=w446:errorcluster)  [unwired: 17 in]
            }
          }
          n173 = call "BaseProcess.set event status.vi"("i ref in"=w422, "EventStatus"=w421, "error in (no error)"=w423) -> ("i ref out"=w430:refnum<vi>, "error out"=w428:errorcluster)  [unwired: 14 in, 1 out]
          n174 = Unbundle By Name(w428) -> ("code"=w432:i32)
          n175 = case shown="No Error" w428 {
            selector: w428 -> [_ w452]
            tunnel: [T3 [] ("byteArray out") w450] -> w429
            frame No Error {
            }
            frame Error {
              n176 = Unbundle By Name(w452) -> ("source"=w451:string)
              n177 = call-poly "CoreLib.data 2 byte array.vi"("string"=w451) -> ("byteArray out"=w450:T3)  [unwired: 18 in]
            }
          }
          n178 = Bundle By Name(cluster=w426, "Data"=w429, "Error #"=w432, "Selector"="C:N") -> (w431:T1)
        }
        frame "Config Keypad and Display" {
          n179 = Unbundle By Name(w470) -> ("Data"=w464:T3)
          n180 = call-poly "CoreLib.byte array 2 data.vi"("byteArray"=w464) -> ("byteArray out"=w461:T3, "i16"=w458:i16, "error out"=w463:errorcluster)  [unwired: 16 in]
          n181 = call-poly "CoreLib.byte array 2 data.vi"("byteArray"=w461, "error in (no error)"=w463) -> ("byteArray out"=w456:T3, "d64"=w462:dbl, "error out"=w457:errorcluster)  [unwired: 15 in]
          n182 = call-poly "CoreLib.byte array 2 data.vi"("byteArray"=w456, "error in (no error)"=w457) -> ("byteArray out"=w455:T3, "i16"=w453:i16, "error out"=w454:errorcluster)  [unwired: 15 in]
          n183 = call-poly "CoreLib.byte array 2 data.vi"("byteArray"=w455, "error in (no error)"=w454) -> ("d64"=w459:dbl, "error out"=w460:errorcluster)  [unwired: 15 in, 1 out]
          n184 = case shown="No Error" w460 {
            tunnel: [w479 w495] -> w466
            tunnel: w468 -> [w491 w495]
            tunnel: w469 -> [w490 w494]
            tunnel: [w478 w493] -> w467
            tunnel: w465 -> [_ w492]
            tunnel: w462 -> [w487 _]
            tunnel: w459 -> [w484 _]
            tunnel: w458 -> [w486 _]
            tunnel: w453 -> [w483 _]
            frame No Error {
              n185 = Greater Than 0?(x=w486) -> (x > 0?=w485:bool)
              n186 = Greater Than 0?(x=w483) -> (x > 0?=w482:bool)
              n187 = call "BNC555.get i attribute.vi"("i ref in"=w491, "error in (no error)"=w490) -> ("i ref out"=w480:refnum<vi>, "i attribute"=w489:T6, "error out"=w481:errorcluster)  [unwired: 15 in]
              n188 = Unbundle By Name(w489) -> ("Information.VISA resource name"=w488:refnum<visa-resource-name>)
              n189 = call "BNC555 Config Keypad & Display.vi"("VISA resource"=w488, "Key Beep (T:On)"=w485, "Beeper Volume (0.1)"=w487, "error in (no error)"=w481, "Key Lock (T:Unlocked)"=w482, "Display Intensity (0.25)"=w484) -> ("error out"=w477:errorcluster)  [unwired: 8 in, 1 out]
              n190 = call "BNC555.HandleError.vi"("i ref in"=w480, "Device error"=w477, "error in (no error)"=w481) -> ("i ref out"=w479:refnum<vi>, "error out"=w478:errorcluster)  [unwired: 15 in]
            }
            frame Error {
              n191 = call "CoreLib.set data type mismatch.vi"("error in (no error)"=w494, "error source"=w492) -> ("error out"=w493:errorcluster)  [unwired: 17 in]
            }
          }
          n192 = call "BaseProcess.set event status.vi"("i ref in"=w466, "EventStatus"=w465, "error in (no error)"=w467) -> ("i ref out"=w474:refnum<vi>, "error out"=w472:errorcluster)  [unwired: 14 in, 1 out]
          n193 = Unbundle By Name(w472) -> ("code"=w476:i32)
          n194 = case shown="No Error" w472 {
            selector: w472 -> [_ w499]
            tunnel: [T3 [] ("byteArray out") w497] -> w473
            frame No Error {
            }
            frame Error {
              n195 = Unbundle By Name(w499) -> ("source"=w498:string)
              n196 = call-poly "CoreLib.data 2 byte array.vi"("string"=w498) -> ("byteArray out"=w497:T3)  [unwired: 18 in]
            }
          }
          n197 = Bundle By Name(cluster=w470, "Data"=w473, "Error #"=w476, "Selector"="C:N") -> (w475:T1)
        }
        frame "Run or Stop" {
          n198 = Unbundle By Name(w508) -> ("Data"=w502:T3)
          n199 = call-poly "CoreLib.byte array 2 data.vi"("byteArray"=w502) -> ("i16"=w501:i16, "error out"=w500:errorcluster)  [unwired: 16 in, 1 out]
          n200 = case shown="No Error" w500 {
            tunnel: [w519 w525] -> w504
            tunnel: w506 -> [w515 w525]
            tunnel: w507 -> [w516 w524]
            tunnel: [w520 w523] -> w505
            tunnel: w503 -> [_ w522]
            tunnel: w501 -> [w521 _]
            frame No Error {
              n201 = Greater Than 0?(x=w521) -> (x > 0?=w517:bool)
              n202 = call "BNC555.Read Sys To Parameters.vi"("i ref in"=w515, "Parameter"=T4."State", "Sys State"=w517, "error in (no error)"=w516) -> ("i ref out"=w519:refnum<vi>, "error out"=w520:errorcluster)  [unwired: 14 in]
            }
            frame Error {
              n203 = call "CoreLib.set data type mismatch.vi"("error in (no error)"=w524, "error source"=w522) -> ("error out"=w523:errorcluster)  [unwired: 17 in]
            }
          }
          n204 = call "BaseProcess.set event status.vi"("i ref in"=w504, "EventStatus"=w503, "error in (no error)"=w505) -> ("i ref out"=w512:refnum<vi>, "error out"=w510:errorcluster)  [unwired: 14 in, 1 out]
          n205 = Unbundle By Name(w510) -> ("code"=w514:i32)
          n206 = case shown="No Error" w510 {
            selector: w510 -> [_ w529]
            tunnel: [T3 [] ("byteArray out") w527] -> w511
            frame No Error {
            }
            frame Error {
              n207 = Unbundle By Name(w529) -> ("source"=w528:string)
              n208 = call-poly "CoreLib.data 2 byte array.vi"("string"=w528) -> ("byteArray out"=w527:T3)  [unwired: 18 in]
            }
          }
          n209 = Bundle By Name(cluster=w508, "Data"=w511, "Error #"=w514, "Selector"="C:N") -> (w513:T1)
        }
        frame "Send SW Trigger" {
          n210 = call "BNC555.get i attribute.vi"("i ref in"=w538, "error in (no error)"=w539) -> ("i ref out"=w533:refnum<vi>, "i attribute"=w536:T6, "error out"=w534:errorcluster)  [unwired: 15 in]
          n211 = Unbundle By Name(w536) -> ("Information.VISA resource name"=w535:refnum<visa-resource-name>)
          n212 = call "BNC555 Send SW Trigger.vi"("VISA resource"=w535, "error in (no error)"=w534) -> ("error out"=w530:errorcluster)  [unwired: 12 in, 1 out]
          n213 = call "BNC555.HandleError.vi"("i ref in"=w533, "Device error"=w530, "error in (no error)"=w534) -> ("i ref out"=w532:refnum<vi>, "error out"=w531:errorcluster)  [unwired: 15 in]
          n214 = call "BaseProcess.set event status.vi"("i ref in"=w532, "EventStatus"=w537, "error in (no error)"=w531) -> ("i ref out"=w544:refnum<vi>, "error out"=w542:errorcluster)  [unwired: 14 in, 1 out]
          n215 = Unbundle By Name(w542) -> ("code"=w546:i32)
          n216 = case shown="No Error" w542 {
            selector: w542 -> [_ w550]
            tunnel: [T3 [] ("byteArray out") w548] -> w543
            frame No Error {
            }
            frame Error {
              n217 = Unbundle By Name(w550) -> ("source"=w549:string)
              n218 = call-poly "CoreLib.data 2 byte array.vi"("string"=w549) -> ("byteArray out"=w548:T3)  [unwired: 18 in]
            }
          }
          n219 = Bundle By Name(cluster=w540, "Data"=w543, "Error #"=w546, "Selector"="C:N") -> (w545:T1)
        }
        frame "Read Sys (To) Parameters" {
          n220 = call "BNC555.get i attribute.vi"("i ref in"=w556, "error in (no error)"=w554) -> ("i ref out"=w555:refnum<vi>, "i attribute"=w552:T6, "error out"=w553:errorcluster)  [unwired: 15 in]
          n221 = Unbundle By Name(w552) -> ("System.Sys State"=w551:bool)
          n222 = call "BNC555.Read Sys To Parameters.vi"("i ref in"=w555, "Parameter"=T4."All Info", "Sys State"=w551, "error in (no error)"=w553) -> ("i ref out"=w559:refnum<vi>, "error out"=w558:errorcluster)  [unwired: 14 in]
          n223 = call "BaseProcess.set event status.vi"("i ref in"=w559, "EventStatus"=w560, "error in (no error)"=w558) -> ("i ref out"=w565:refnum<vi>, "error out"=w563:errorcluster)  [unwired: 14 in, 1 out]
          n224 = Unbundle By Name(w563) -> ("code"=w567:i32)
          n225 = case shown="No Error" w563 {
            selector: w563 -> [_ w571]
            tunnel: [T3 [] ("byteArray out") w569] -> w564
            frame No Error {
            }
            frame Error {
              n226 = Unbundle By Name(w571) -> ("source"=w570:string)
              n227 = call-poly "CoreLib.data 2 byte array.vi"("string"=w570) -> ("byteArray out"=w569:T3)  [unwired: 18 in]
            }
          }
          n228 = Bundle By Name(cluster=w561, "Data"=w564, "Error #"=w567, "Selector"="C:N") -> (w566:T1)
        }
        frame "Chan On or Off" {
          n229 = Unbundle By Name(w575) -> ("Data"=w583:T3)
          n230 = call-poly "CoreLib.byte array 2 data.vi"("byteArray"=w583) -> ("byteArray out"=w579:T3, "i32"=w582:i32, "error out"=w581:errorcluster)  [unwired: 16 in]
          n231 = call-poly "CoreLib.byte array 2 data.vi"("byteArray"=w579, "error in (no error)"=w581) -> ("i16"=w580:i16, "error out"=w578:errorcluster)  [unwired: 15 in, 1 out]
          n232 = case shown="No Error" w578 {
            tunnel: [w597 w605] -> w574
            tunnel: w577 -> [w601 w605]
            tunnel: w576 -> [w600 w604]
            tunnel: [w596 w603] -> w573
            tunnel: w572 -> [_ w602]
            tunnel: w582 -> [w592 _]
            tunnel: w580 -> [w593 _]
            frame No Error {
              n233 = Greater Than 0?(x=w593) -> (x > 0?=w591:bool)
              n234 = call "BNC555.get i attribute.vi"("i ref in"=w601, "error in (no error)"=w600) -> ("i ref out"=w598:refnum<vi>, "i attribute"=w599:T6, "error out"=w594:errorcluster)  [unwired: 15 in]
              n235 = Unbundle By Name(w599) -> ("Information.VISA resource name"=w595:refnum<visa-resource-name>)
              n236 = call "BNC555 Chan On_Off.vi"("VISA resource"=w595, "Channel (1:Chan A)"=w592, "State (T:On)"=w591, "error in (no error)"=w594) -> ()  [unwired: 10 in, 2 out]
              n237 = call "BNC555.Read Channel Parameters.vi"("i ref in"=w598, "Channel (1: Chan A)"=w592, "Parameter"=T5."State (On/Off)", "error in (no error)"=w594) -> ("i ref out"=w597:refnum<vi>, "error out"=w596:errorcluster)  [unwired: 14 in]
            }
            frame Error {
              n238 = call "CoreLib.set data type mismatch.vi"("error in (no error)"=w604, "error source"=w602) -> ("error out"=w603:errorcluster)  [unwired: 17 in]
            }
          }
          n239 = call "BaseProcess.set event status.vi"("i ref in"=w574, "EventStatus"=w572, "error in (no error)"=w573) -> ("i ref out"=w587:refnum<vi>, "error out"=w585:errorcluster)  [unwired: 14 in, 1 out]
          n240 = Unbundle By Name(w585) -> ("code"=w589:i32)
          n241 = case shown="No Error" w585 {
            selector: w585 -> [_ w609]
            tunnel: [T3 [] ("byteArray out") w607] -> w586
            frame No Error {
            }
            frame Error {
              n242 = Unbundle By Name(w609) -> ("source"=w608:string)
              n243 = call-poly "CoreLib.data 2 byte array.vi"("string"=w608) -> ("byteArray out"=w607:T3)  [unwired: 18 in]
            }
          }
          n244 = Bundle By Name(cluster=w575, "Data"=w586, "Error #"=w589, "Selector"="C:N") -> (w588:T1)
        }
        frame "Chan Gating On or Off" {
          n245 = Unbundle By Name(w613) -> ("Data"=w621:T3)
          n246 = call-poly "CoreLib.byte array 2 data.vi"("byteArray"=w621) -> ("byteArray out"=w617:T3, "i32"=w620:i32, "error out"=w619:errorcluster)  [unwired: 16 in]
          n247 = call-poly "CoreLib.byte array 2 data.vi"("byteArray"=w617, "error in (no error)"=w619) -> ("i16"=w618:i16, "error out"=w616:errorcluster)  [unwired: 15 in, 1 out]
          n248 = case shown="No Error" w616 {
            tunnel: [w635 w643] -> w612
            tunnel: w615 -> [w639 w643]
            tunnel: w614 -> [w638 w642]
            tunnel: [w634 w641] -> w611
            tunnel: w610 -> [_ w640]
            tunnel: w620 -> [w629 _]
            tunnel: w618 -> [w633 _]
            frame No Error {
              n249 = Greater Than 0?(x=w633) -> (x > 0?=w630:bool)
              n250 = call "BNC555.get i attribute.vi"("i ref in"=w639, "error in (no error)"=w638) -> ("i ref out"=w636:refnum<vi>, "i attribute"=w637:T6, "error out"=w631:errorcluster)  [unwired: 15 in]
              n251 = Unbundle By Name(w637) -> ("Information.VISA resource name"=w632:refnum<visa-resource-name>)
              n252 = call "BNC555 Chan Gating On_Off.vi"("VISA resource"=w632, "Channel (1:Chan A)"=w629, "State (F:Off)"=w630, "error in (no error)"=w631) -> ()  [unwired: 10 in, 2 out]
              n253 = call "BNC555.Read Channel Parameters.vi"("i ref in"=w636, "Channel (1: Chan A)"=w629, "Parameter"=T5."Gate Config", "error in (no error)"=w631) -> ("i ref out"=w635:refnum<vi>, "error out"=w634:errorcluster)  [unwired: 14 in]
            }
            frame Error {
              n254 = call "CoreLib.set data type mismatch.vi"("error in (no error)"=w642, "error source"=w640) -> ("error out"=w641:errorcluster)  [unwired: 17 in]
            }
          }
          n255 = call "BaseProcess.set event status.vi"("i ref in"=w612, "EventStatus"=w610, "error in (no error)"=w611) -> ("i ref out"=w625:refnum<vi>, "error out"=w623:errorcluster)  [unwired: 14 in, 1 out]
          n256 = Unbundle By Name(w623) -> ("code"=w627:i32)
          n257 = case shown="No Error" w623 {
            selector: w623 -> [_ w647]
            tunnel: [T3 [] ("byteArray out") w645] -> w624
            frame No Error {
            }
            frame Error {
              n258 = Unbundle By Name(w647) -> ("source"=w646:string)
              n259 = call-poly "CoreLib.data 2 byte array.vi"("string"=w646) -> ("byteArray out"=w645:T3)  [unwired: 18 in]
            }
          }
          n260 = Bundle By Name(cluster=w613, "Data"=w624, "Error #"=w627, "Selector"="C:N") -> (w626:T1)
        }
        frame "Read Chan Parameters" {
          n261 = call "BNC555.get i attribute.vi"("i ref in"=w658, "error in (no error)"=w657) -> ("i ref out"=w651:refnum<vi>, "i attribute"=w652:T6, "error out"=w650:errorcluster)  [unwired: 15 in]
          n262 = Unbundle By Name(w652) -> ("Channel Array"=w649:T7[])
          n263 = for {
            tunnel: w649 -> [w667] mode=indexing
            shift-right: [w670] -> w654
            shift-left: w650 -> [w668]
            shift-right: [w671] -> w655
            shift-left: w651 -> [w669]
            tunnel: T5."All Info" ("Parameter") -> [w665]
            n264 = Unbundle By Name(w667) -> ("Chan #"=w666:i32)
            n265 = call "BNC555.Read Channel Parameters.vi"("i ref in"=w669, "Channel (1: Chan A)"=w666, "Parameter"=w665, "error in (no error)"=w668) -> ("i ref out"=w671:refnum<vi>, "error out"=w670:errorcluster)  [unwired: 14 in]
          }
          n266 = call "BaseProcess.set event status.vi"("i ref in"=w655, "EventStatus"=w653, "error in (no error)"=w654) -> ("i ref out"=w662:refnum<vi>, "error out"=w660:errorcluster)  [unwired: 14 in, 1 out]
          n267 = Unbundle By Name(w660) -> ("code"=w664:i32)
          n268 = case shown="No Error" w660 {
            selector: w660 -> [_ w675]
            tunnel: [T3 [] ("byteArray out") w673] -> w661
            frame No Error {
            }
            frame Error {
              n269 = Unbundle By Name(w675) -> ("source"=w674:string)
              n270 = call-poly "CoreLib.data 2 byte array.vi"("string"=w674) -> ("byteArray out"=w673:T3)  [unwired: 18 in]
            }
          }
          n271 = Bundle By Name(cluster=w656, "Data"=w661, "Error #"=w664, "Selector"="C:N") -> (w663:T1)
        }
        frame "Read or Save Memory" {
          n272 = Unbundle By Name(w680) -> ("Data"=w677:T3)
          n273 = call-poly "CoreLib.byte array 2 data.vi"("byteArray"=w677) -> ("byteArray out"=w678:T3, "i32"=w676:i32, "error out"=w679:errorcluster)  [unwired: 16 in]
          n274 = call-poly "CoreLib.byte array 2 data.vi"("byteArray"=w678, "error in (no error)"=w679) -> ("i16"=w687:i16, "error out"=w686:errorcluster)  [unwired: 15 in, 1 out]
          n275 = case shown="No Error" w686 {
            tunnel: [w699 w709] -> w682
            tunnel: w685 -> [w705 w709]
            tunnel: w684 -> [w704 w708]
            tunnel: [w701 w707] -> w683
            tunnel: w681 -> [_ w706]
            tunnel: w687 -> [w702 _]
            tunnel: w676 -> [w694 _]
            frame No Error {
              n276 = Greater Than 0?(x=w702) -> (x > 0?=w696:bool)
              n277 = call "BNC555.get i attribute.vi"("i ref in"=w705, "error in (no error)"=w704) -> ("i ref out"=w700:refnum<vi>, "i attribute"=w703:T6, "error out"=w698:errorcluster)  [unwired: 15 in]
              n278 = Unbundle By Name(w703) -> ("Information.VISA resource name"=w695:refnum<visa-resource-name>)
              n279 = call "BNC555 Read_Save Memory.vi"("VISA resource"=w695, "Memory  (1)"=w694, "Read/Save (F:Read)"=w696, "error in (no error)"=w698) -> ("error out"=w697:errorcluster)  [unwired: 10 in, 1 out]
              n280 = call "BNC555.HandleError.vi"("i ref in"=w700, "Device error"=w697, "error in (no error)"=w698) -> ("i ref out"=w699:refnum<vi>, "error out"=w701:errorcluster)  [unwired: 15 in]
            }
            frame Error {
              n281 = call "CoreLib.set data type mismatch.vi"("error in (no error)"=w708, "error source"=w706) -> ("error out"=w707:errorcluster)  [unwired: 17 in]
            }
          }
          n282 = call "BaseProcess.set event status.vi"("i ref in"=w682, "EventStatus"=w681, "error in (no error)"=w683) -> ("i ref out"=w691:refnum<vi>, "error out"=w689:errorcluster)  [unwired: 14 in, 1 out]
          n283 = Unbundle By Name(w689) -> ("code"=w693:i32)
          n284 = case shown="No Error" w689 {
            selector: w689 -> [_ w713]
            tunnel: [T3 [] ("byteArray out") w711] -> w690
            frame No Error {
            }
            frame Error {
              n285 = Unbundle By Name(w713) -> ("source"=w712:string)
              n286 = call-poly "CoreLib.data 2 byte array.vi"("string"=w712) -> ("byteArray out"=w711:T3)  [unwired: 18 in]
            }
          }
          n287 = Bundle By Name(cluster=w680, "Data"=w690, "Error #"=w693, "Selector"="C:N") -> (w692:T1)
        }
        frame "Self-Test" {
          n288 = call "BNC555.Self-Test.vi"("i ref in"=w719, "error IO"=w718) -> ("i ref out"=w716:refnum<vi>, "error out"=w717:errorcluster)  [unwired: 16 in]
          n289 = call "BaseProcess.set event status.vi"("i ref in"=w716, "EventStatus"=w715, "error in (no error)"=w717) -> ("i ref out"=w723:refnum<vi>, "error out"=w721:errorcluster)  [unwired: 14 in, 1 out]
          n290 = Unbundle By Name(w721) -> ("code"=w725:i32)
          n291 = case shown="No Error" w721 {
            selector: w721 -> [_ w729]
            tunnel: [T3 [] ("byteArray out") w727] -> w722
            frame No Error {
            }
            frame Error {
              n292 = Unbundle By Name(w729) -> ("source"=w728:string)
              n293 = call-poly "CoreLib.data 2 byte array.vi"("string"=w728) -> ("byteArray out"=w727:T3)  [unwired: 18 in]
            }
          }
          n294 = Bundle By Name(cluster=w714, "Data"=w722, "Error #"=w725, "Selector"="C:N") -> (w724:T1)
        }
        frame "Revision Query" {
          n295 = call "BNC555.Revision Query.vi"("i ref in"=w735, "error IO"=w734) -> ("i ref out"=w732:refnum<vi>, "error out"=w733:errorcluster)  [unwired: 16 in]
          n296 = call "BaseProcess.set event status.vi"("i ref in"=w732, "EventStatus"=w731, "error in (no error)"=w733) -> ("i ref out"=w739:refnum<vi>, "error out"=w737:errorcluster)  [unwired: 14 in, 1 out]
          n297 = Unbundle By Name(w737) -> ("code"=w741:i32)
          n298 = case shown="No Error" w737 {
            selector: w737 -> [_ w745]
            tunnel: [T3 [] ("byteArray out") w743] -> w738
            frame No Error {
            }
            frame Error {
              n299 = Unbundle By Name(w745) -> ("source"=w744:string)
              n300 = call-poly "CoreLib.data 2 byte array.vi"("string"=w744) -> ("byteArray out"=w743:T3)  [unwired: 18 in]
            }
          }
          n301 = Bundle By Name(cluster=w730, "Data"=w738, "Error #"=w741, "Selector"="C:N") -> (w740:T1)
        }
        frame "Reset" {
          n302 = call "BNC555.Reset.vi"("i ref in"=w749, "error IO"=w747) -> ("i ref out"=w748:refnum<vi>, "error out"=w746:errorcluster)  [unwired: 16 in]
          n303 = call "BaseProcess.set event status.vi"("i ref in"=w748, "EventStatus"=w751, "error in (no error)"=w746) -> ("i ref out"=w755:refnum<vi>, "error out"=w753:errorcluster)  [unwired: 14 in, 1 out]
          n304 = Unbundle By Name(w753) -> ("code"=w757:i32)
          n305 = case shown="No Error" w753 {
            selector: w753 -> [_ w761]
            tunnel: [T3 [] ("byteArray out") w759] -> w754
            frame No Error {
            }
            frame Error {
              n306 = Unbundle By Name(w761) -> ("source"=w760:string)
              n307 = call-poly "CoreLib.data 2 byte array.vi"("string"=w760) -> ("byteArray out"=w759:T3)  [unwired: 18 in]
            }
          }
          n308 = Bundle By Name(cluster=w750, "Data"=w754, "Error #"=w757, "Selector"="C:N") -> (w756:T1)
        }
        frame "_set_PSDB_Data" {
          n309 = call "CAEObj.unfold trend data.vi"("i ref in"=w765, "raw trend data"=w762) -> ("quality"=w767:i32, "no link"=w770:bool, "data"=w768:i8[], "typeDescriptor"=w769:string, "error out"=w771:errorcluster)  [unwired: 9 in, 4 out]
          n310 = case shown="No Error" w771 {
            tunnel: w766 -> [w791 w801]
            tunnel: [w790 w800] -> w763
            tunnel: [w789 w801] -> w764
            tunnel: w765 -> [w787 w800]
            tunnel: w770 -> [w781 _]
            tunnel: w769 -> [w783 _]
            tunnel: w768 -> [w784 _]
            tunnel: w767 -> [w782 _]
            frame No Error {
              n311 = call "PH_PSDBWriter.get Subsystem DIM Service.vi"("no link"=w781, "typeDescriptor"=w783, "data"=w784, "quality"=w782) -> ("PHELIX Subsystems"=w780:T9)
              n312 = call "PH_PSDBWriter.check PSDB writing condition.vi"("i ref in"=w787, "wanted Subsystem"=w780, "error IO"=w791) -> ("i ref out"=w786:refnum<vi>, "write PSDB?"=w785:bool, "error out"=w788:errorcluster)  [unwired: 14 in]
              n313 = case shown="False" w785 {
                tunnel: w788 -> [w792 w799]
                tunnel: [w793 w796] -> w790
                tunnel: [w792 w794] -> w789
                tunnel: w786 -> [w793 w798]
                frame False {
                }
                frame True {
                  n314 = call "BNC555.PC Write PSDB.vi"("i ref in"=w798, "error IO"=w799) -> ("i ref out"=w797:refnum<vi>, "error out"=w795:errorcluster)  [unwired: 16 in]
                  n315 = call "PH_PSDBWriter.evt call write PSDB.vi"("i ref in"=w797, "error in (no error)"=w795) -> ("i ref out"=w796:refnum<vi>, "error out"=w794:errorcluster)  [unwired: 16 in]
                }
              }
            }
            frame Error {
            }
          }
          n316 = call "BaseProcess.set event status.vi"("i ref in"=w763, "EventStatus"=w773, "error in (no error)"=w764) -> ("i ref out"=w777:refnum<vi>, "error out"=w775:errorcluster)  [unwired: 14 in, 1 out]
          n317 = Unbundle By Name(w775) -> ("code"=w779:i32)
          n318 = case shown="No Error" w775 {
            selector: w775 -> [_ w805]
            tunnel: [T3 [] ("byteArray out") w803] -> w776
            frame No Error {
            }
            frame Error {
              n319 = Unbundle By Name(w805) -> ("source"=w804:string)
              n320 = call-poly "CoreLib.data 2 byte array.vi"("string"=w804) -> ("byteArray out"=w803:T3)  [unwired: 18 in]
            }
          }
          n321 = Bundle By Name(cluster=w772, "Data"=w776, "Error #"=w779, "Selector"="C:N") -> (w778:T1)
        }
      }
    }
    frame Error {
    }
  }
  "answer cluster" <- w7
  "i ref out" <- w4
  "error out" <- w3
